vi "Dresden Edit Recipe(in).vi"() -> ()   [LabVIEW 2009] (continued)
                    n928 = local read "R Z_factor"() -> (w1701:dbl)
                    n929 = Equal To 0?(x=w1698) -> (x = 0?=w1697:bool)
                    n930 = Equal To 0?(x=w1701) -> (x = 0?=w1699:bool)
                    n931 = Equal To 0?(x=w1702) -> (x = 0?=w1700:bool)
                  }
                }
                n932 = local read "R Set Pressure mtorr"() -> (w1318:dbl)
                n933 = local read "R Argon Flow sccm"() -> (w1319:dbl)
                n934 = case shown="True" w1178 {
                  tunnel: [FALSE w1396] -> w1183
                  frame #0 {
                  }
                  frame #1 {
                    # "101"
                    n935 = local read "Calculated_total_length_dc"() -> (w1398:dbl)
                    n936 = local read "R  Total length"() -> (w1397:dbl)
                    n937 = Less?(x=w1397, y=w1398) -> (x < y?=w1396:bool)
                  }
                }
                n938 = case shown="True" w1279 {
                  tunnel: [FALSE w1388] -> w1181
                  frame #0 {
                  }
                  frame #1 {
                    # "103"
                    n939 = local read "Calculated_total_length_cmb"() -> (w1390:dbl)
                    n940 = local read "R  Total length"() -> (w1389:dbl)
                    n941 = Less?(x=w1389, y=w1390) -> (x < y?=w1388:bool)
                  }
                }
                n942 = case shown="True" w1180 {
                  tunnel: [FALSE w1392] -> w1182
                  frame #0 {
                  }
                  frame #1 {
                    # "102"
                    n943 = local read "Calculated_total_length_rf"() -> (w1394:dbl)
                    n944 = local read "R  Total length"() -> (w1393:dbl)
                    n945 = Less?(x=w1393, y=w1394) -> (x < y?=w1392:bool)
                  }
                }
                n946 = Equal To 0?(x=w1318) -> (x = 0?=w1191:bool)
                n947 = Equal To 0?(x=w1319) -> (x = 0?=w1192:bool)
                n948 = Build Array(FALSE, w1349, w1314, w1317, w1316, w1307, w1315, w1278, w1277, w1276, w1275, w1274, w1273, w1272, w1271, w1270, w1269, w1268, w1267, w1266, w1265, w1264, w1263, w1262, w1261, w1260, w1259, w1258, w1257, w1256, w1252, w1251, w1250, w1249, w1248, w1247, w1246, w1245, w1244, w1243, w1242, w1241, w1240, w1239, w1238, w1237, w1236, w1235, w1234, w1233, w1232, w1231, w1230, w1229, w1228, w1227, w1226, w1225, w1224, w1223, w1222, w1221, w1220, w1219, w1218, w1217, w1216, w1215, w1214, w1213, w1212, w1211, w1210, w1209, w1208, w1207, w1206, w1205, w1204, w1203, w1202, w1201, w1200, w1199, w1198, w1197, w1196, w1195, w1194, w1193, w1192, w1191, w1190, w1189, w1188, w1187, w1186, w1185, w1184, w1162, w1183, w1182, w1181) -> (w1255:bool[])
                n949 = Boolean To (0,1)(Boolean=w1255) -> (0, 1=w1254:i16[])
                n950 = Array Max & Min(array=w1254) -> (max index (indices)=w1253:i32)  [unwired: 3 out]
                n951 = case shown="4" w1253 {
                  tunnel: [TRUE FALSE FALSE FALSE FALSE FALSE FALSE FALSE FALSE FALSE FALSE FALSE FALSE FALSE FALSE FALSE FALSE FALSE FALSE FALSE FALSE FALSE FALSE FALSE FALSE FALSE FALSE FALSE FALSE FALSE FALSE FALSE FALSE FALSE FALSE FALSE FALSE FALSE FALSE FALSE FALSE FALSE FALSE FALSE FALSE FALSE FALSE FALSE FALSE FALSE FALSE FALSE FALSE FALSE FALSE FALSE FALSE FALSE FALSE FALSE FALSE FALSE FALSE FALSE FALSE FALSE FALSE FALSE FALSE FALSE FALSE FALSE FALSE FALSE FALSE FALSE FALSE FALSE FALSE FALSE FALSE FALSE FALSE FALSE FALSE FALSE FALSE FALSE FALSE FALSE FALSE FALSE FALSE FALSE FALSE FALSE FALSE FALSE FALSE FALSE FALSE FALSE FALSE FALSE] -> w1310
                  frame #0 {
                  }
                  frame #1 {
                    n952 = One Button Dialog(message="Please enter the Recipe name !") -> ()  [unwired: 1 in, 1 out]
                  }
                  frame #2 {
                    n953 = One Button Dialog(message="Please enter the Substrate Material name !") -> ()  [unwired: 1 in, 1 out]
                  }
                  frame #3 {
                    n954 = One Button Dialog(message="Please enter Microwave Power!") -> ()  [unwired: 1 in, 1 out]
                  }
                  frame #4 {
                    n955 = One Button Dialog(message="Please enter Pass Number !") -> ()  [unwired: 1 in, 1 out]
                  }
                  frame #5 {
                    n956 = One Button Dialog(message="Please enter Microwave Duration !") -> ()  [unwired: 1 in, 1 out]
                  }
                  frame #6 {
                    n957 = One Button Dialog(message="Please enter DC Target Material name !") -> ()  [unwired: 1 in, 1 out]
                  }
                  frame #7 {
                    n958 = One Button Dialog(message="Please click Process List!") -> ()  [unwired: 1 in, 1 out]
                  }
                  frame #8 {
                    n959 = One Button Dialog(message="Please enter DC Coating Power!") -> ()  [unwired: 1 in, 1 out]
                  }
                  frame #9 {
                    n960 = One Button Dialog(message="Please enter interval length!") -> ()  [unwired: 1 in, 1 out]
                  }
                  frame #10 {
                    n961 = One Button Dialog(message="Please enter DC Coating Power!") -> ()  [unwired: 1 in, 1 out]
                  }
                  frame #11 {
                    n962 = One Button Dialog(message="Please enter interval length!") -> ()  [unwired: 1 in, 1 out]
                  }
                  frame #12 {
                    n963 = One Button Dialog(message="Please enter DC Coating Power !") -> ()  [unwired: 1 in, 1 out]
                  }
                  frame #13 {
                    n964 = One Button Dialog(message="Please enter interval length!") -> ()  [unwired: 1 in, 1 out]
                  }
                  frame #14 {
                    n965 = One Button Dialog(message="Please enter DC Coating Power!") -> ()  [unwired: 1 in, 1 out]
                  }
                  frame #15 {
                    n966 = One Button Dialog(message="Please enter interval length!") -> ()  [unwired: 1 in, 1 out]
                  }
                  frame #16 {
                    n967 = One Button Dialog(message="Please enter DC Coating Power !") -> ()  [unwired: 1 in, 1 out]
                  }
                  frame #17 {
                    n968 = One Button Dialog(message="Please enter interval length!") -> ()  [unwired: 1 in, 1 out]
                  }
                  frame #18 {
                    n969 = One Button Dialog(message="Please enter DC Coating Power !") -> ()  [unwired: 1 in, 1 out]
                  }
                  frame #19 {
                    n970 = One Button Dialog(message="Please enter interval length!") -> ()  [unwired: 1 in, 1 out]
                  }
                  frame #20 {
                    n971 = One Button Dialog(message="Please enter DC Coating Power !") -> ()  [unwired: 1 in, 1 out]
                  }
                  frame #21 {
                    n972 = One Button Dialog(message="Please enter interval length!") -> ()  [unwired: 1 in, 1 out]
                  }
                  frame #22 {
                    n973 = One Button Dialog(message="Please enter DC Coating Power !") -> ()  [unwired: 1 in, 1 out]
                  }
                  frame #23 {
                    n974 = One Button Dialog(message="Please enter interval length!") -> ()  [unwired: 1 in, 1 out]
                  }
                  frame #24 {
                    n975 = One Button Dialog(message="Please enter DC Coating Power !") -> ()  [unwired: 1 in, 1 out]
                  }
                  frame #25 {
                    n976 = One Button Dialog(message="Please enter interval length!") -> ()  [unwired: 1 in, 1 out]
                  }
                  frame #26 {
                    n977 = One Button Dialog(message="Please enter DC Coating Power !") -> ()  [unwired: 1 in, 1 out]
                  }
                  frame #27 {
                    n978 = One Button Dialog(message="Please enter interval length!") -> ()  [unwired: 1 in, 1 out]
                  }
                  frame #28 {
                    n979 = One Button Dialog(message="Please enter RF Target Material !") -> ()  [unwired: 1 in, 1 out]
                  }
                  frame #29 {
                    n980 = One Button Dialog(message="Please click Process List!") -> ()  [unwired: 1 in, 1 out]
                  }
                  frame #30 {
                    n981 = One Button Dialog(message="Please enter RF Ramp Up Time!") -> ()  [unwired: 1 in, 1 out]
                  }
                  frame #31 {
                    n982 = One Button Dialog(message="Please enter RF Coating Power  !") -> ()  [unwired: 1 in, 1 out]
                  }
                  frame #32 {
                    n983 = One Button Dialog(message="Please enter interval length !") -> ()  [unwired: 1 in, 1 out]
                  }
                  frame #33 {
                    n984 = One Button Dialog(message="Please enter RF Coating Power  !") -> ()  [unwired: 1 in, 1 out]
                  }
                  frame #34 {
                    n985 = One Button Dialog(message="Please enter interval length!") -> ()  [unwired: 1 in, 1 out]
                  }
                  frame #35 {
                    n986 = One Button Dialog(message="Please enter RF Coating Power  !") -> ()  [unwired: 1 in, 1 out]
                  }
                  frame #36 {
                    n987 = One Button Dialog(message="Please enter interval length!") -> ()  [unwired: 1 in, 1 out]
                  }
                  frame #37 {
                    n988 = One Button Dialog(message="Please enter RF Coating Power !") -> ()  [unwired: 1 in, 1 out]
                  }
                  frame #38 {
                    n989 = One Button Dialog(message="Please enter interval length!") -> ()  [unwired: 1 in, 1 out]
                  }
                  frame #39 {
                    n990 = One Button Dialog(message="Please enter RF Coating Power !") -> ()  [unwired: 1 in, 1 out]
                  }
                  frame #40 {
                    n991 = One Button Dialog(message="Please enter interval length!") -> ()  [unwired: 1 in, 1 out]
                  }
                  frame #41 {
                    n992 = One Button Dialog(message="Please enter RF Coating Power !") -> ()  [unwired: 1 in, 1 out]
                  }
                  frame #42 {
                    n993 = One Button Dialog(message="Please enter interval length!") -> ()  [unwired: 1 in, 1 out]
                  }
                  frame #43 {
                    n994 = One Button Dialog(message="Please enter RF Coating Power !") -> ()  [unwired: 1 in, 1 out]
                  }
                  frame #44 {
                    n995 = One Button Dialog(message="Please enter interval length!") -> ()  [unwired: 1 in, 1 out]
                  }
                  frame #45 {
                    n996 = One Button Dialog(message="Please enter RF Coating Power !") -> ()  [unwired: 1 in, 1 out]
                  }
                  frame #46 {
                    n997 = One Button Dialog(message="Please enter interval length!") -> ()  [unwired: 1 in, 1 out]
                  }
                  frame #47 {
                    n998 = One Button Dialog(message="Please enter RF Coating Power !") -> ()  [unwired: 1 in, 1 out]
                  }
                  frame #48 {
                    n999 = One Button Dialog(message="Please enter interval length!") -> ()  [unwired: 1 in, 1 out]
                  }
                  frame #49 {
                    n1000 = One Button Dialog(message="Please enter RF Coating Power !") -> ()  [unwired: 1 in, 1 out]
                  }
                  frame #50 {
                    n1001 = One Button Dialog(message="Please enter interval length!") -> ()  [unwired: 1 in, 1 out]
                  }
                  frame #51 {
                    n1002 = One Button Dialog(message="Please enter RF Ramp Down Time  !") -> ()  [unwired: 1 in, 1 out]
                  }
                  frame #52 {
                    n1003 = One Button Dialog(message="Please enter Chamber II\nTarget Material name!") -> ()  [unwired: 1 in, 1 out]
                  }
                  frame #53 {
                    n1004 = One Button Dialog(message="Please enter web speed!") -> ()  [unwired: 1 in, 1 out]
                  }
                  frame #54 {
                    n1005 = One Button Dialog(message="Please enter Chamber III Target Material \nName !") -> ()  [unwired: 1 in, 1 out]
                  }
                  frame #55 {
                    n1006 = One Button Dialog(message="Please enter Web Speed !") -> ()  [unwired: 1 in, 1 out]
                  }
                  frame #56 {
                    n1007 = One Button Dialog(message="Please click process list !") -> ()  [unwired: 1 in, 1 out]
                  }
                  frame #57 {
                    n1008 = One Button Dialog(message="Please enter Number of Cycle !") -> ()  [unwired: 1 in, 1 out]
                  }
                  frame #58 {
                    n1009 = One Button Dialog(message="Please enter Chamber II  Coating Power !") -> ()  [unwired: 1 in, 1 out]
                  }
                  frame #59 {
                    n1010 = One Button Dialog(message="Please enter Chamber III  Coating Power !") -> ()  [unwired: 1 in, 1 out]
                  }
                  frame #60 {
                    n1011 = One Button Dialog(message="Please enter interval length!") -> ()  [unwired: 1 in, 1 out]
                  }
                  frame #61 {
                    n1012 = One Button Dialog(message="Please enter Chamber II  Coating Power !") -> ()  [unwired: 1 in, 1 out]
                  }
                  frame #62 {
                    n1013 = One Button Dialog(message="Please enter Chamber III  Coating Power !") -> ()  [unwired: 1 in, 1 out]
                  }
                  frame #63 {
                    n1014 = One Button Dialog(message="Please enter interval length!") -> ()  [unwired: 1 in, 1 out]
                  }
                  frame #64 {
                    n1015 = One Button Dialog(message="Please enter Chamber II  Coating Power !") -> ()  [unwired: 1 in, 1 out]
                  }
                  frame #65 {
                    n1016 = One Button Dialog(message="Please enter Chamber III Coating Power !") -> ()  [unwired: 1 in, 1 out]
                  }
                  frame #66 {
                    n1017 = One Button Dialog(message="Please enter interval length!") -> ()  [unwired: 1 in, 1 out]
                  }
                  frame #67 {
                    n1018 = One Button Dialog(message="Please enter Chamber II  Coating Power !") -> ()  [unwired: 1 in, 1 out]
                  }
                  frame #68 {
                    n1019 = One Button Dialog(message="Please enter Chamber III  Coating Power !") -> ()  [unwired: 1 in, 1 out]
                  }
                  frame #69 {
                    n1020 = One Button Dialog(message="Please enter interval length!") -> ()  [unwired: 1 in, 1 out]
                  }
                  frame #70 {
                    n1021 = One Button Dialog(message="Please enter Chamber II  Coating Power !") -> ()  [unwired: 1 in, 1 out]
                  }
                  frame #71 {
                    n1022 = One Button Dialog(message="Please enter Chamber III  Coating Power !") -> ()  [unwired: 1 in, 1 out]
                  }
                  frame #72 {
                    n1023 = One Button Dialog(message="Please enter interval length!") -> ()  [unwired: 1 in, 1 out]
                  }
                  frame #73 {
                    n1024 = One Button Dialog(message="Please enter Chamber II  Coating Power !") -> ()  [unwired: 1 in, 1 out]
                  }
                  frame #74 {
                    n1025 = One Button Dialog(message="Please enter Chamber III  Coating Power !") -> ()  [unwired: 1 in, 1 out]
                  }
                  frame #75 {
                    n1026 = One Button Dialog(message="Please enter interval length!") -> ()  [unwired: 1 in, 1 out]
                  }
                  frame #76 {
                    n1027 = One Button Dialog(message="Please enter Chamber II  Coating Power !") -> ()  [unwired: 1 in, 1 out]
                  }
                  frame #77 {
                    n1028 = One Button Dialog(message="Please enter Chamber III  Coating Power !") -> ()  [unwired: 1 in, 1 out]
                  }
                  frame #78 {
                    n1029 = One Button Dialog(message="Please enter interval length!") -> ()  [unwired: 1 in, 1 out]
                  }
                  frame #79 {
                    n1030 = One Button Dialog(message="Please enter Chamber II  Coating Power !") -> ()  [unwired: 1 in, 1 out]
                  }
                  frame #80 {
                    n1031 = One Button Dialog(message="Please enter Chamber III  Coating Power !") -> ()  [unwired: 1 in, 1 out]
                  }
                  frame #81 {
                    n1032 = One Button Dialog(message="Please enter interval length!") -> ()  [unwired: 1 in, 1 out]
                  }
                  frame #82 {
                    n1033 = One Button Dialog(message="Please enter Chamber II  Coating Power !") -> ()  [unwired: 1 in, 1 out]
                  }
                  frame #83 {
                    n1034 = One Button Dialog(message="Please enter Chamber III  Coating Power !") -> ()  [unwired: 1 in, 1 out]
                  }
                  frame #84 {
                    n1035 = One Button Dialog(message="Please enter interval length!") -> ()  [unwired: 1 in, 1 out]
                  }
                  frame #85 {
                    n1036 = One Button Dialog(message="Please enter Chamber II  Coating Power !") -> ()  [unwired: 1 in, 1 out]
                  }
                  frame #86 {
                    n1037 = One Button Dialog(message="Please enter Chamber III  Coating Power !") -> ()  [unwired: 1 in, 1 out]
                  }
                  frame #87 {
                    n1038 = One Button Dialog(message="Please enter interval length!") -> ()  [unwired: 1 in, 1 out]
                  }
                  frame #88 {
                    n1039 = One Button Dialog(message="Please enter Material Density !") -> ()  [unwired: 1 in, 1 out]
                  }
                  frame #89 {
                    n1040 = One Button Dialog(message="Please enter Z factor !") -> ()  [unwired: 1 in, 1 out]
                  }
                  frame #90 {
                    n1041 = One Button Dialog(message="Please enter Tooling Factor !") -> ()  [unwired: 1 in, 1 out]
                  }
                  frame #91 {
                    n1042 = One Button Dialog(message="Please enter Argon Flow !") -> ()  [unwired: 1 in, 1 out]
                  }
                  frame #92 {
                    n1043 = One Button Dialog(message="Please enter Set Pressure !") -> ()  [unwired: 1 in, 1 out]
                  }
                  frame #93 {
                    n1044 = One Button Dialog(message="Please enter Target thickness Value!") -> ()  [unwired: 1 in, 1 out]
                  }
                  frame #94 {
                    n1045 = One Button Dialog(message="Please enter Duration!") -> ()  [unwired: 1 in, 1 out]
                  }
                  frame #95 {
                    n1046 = One Button Dialog(message="Please enter Minimum Diameter !") -> ()  [unwired: 1 in, 1 out]
                  }
                  frame #96 {
                    n1047 = One Button Dialog(message="Please enter Maximum Diameter !") -> ()  [unwired: 1 in, 1 out]
                  }
                  frame #97 {
                    n1048 = One Button Dialog(message="Please enter Web Speed !") -> ()  [unwired: 1 in, 1 out]
                  }
                  frame #98 {
                    n1049 = One Button Dialog(message="Please enter Web Thickness !") -> ()  [unwired: 1 in, 1 out]
                  }
                  frame #99 {
                    n1050 = One Button Dialog(message="Please enter Tension Value !") -> ()  [unwired: 1 in, 1 out]
                  }
                  frame #100 {
                    n1051 = One Button Dialog(message="Please click equal sign!") -> ()  [unwired: 1 in, 1 out]
                  }
                  frame #101 {
                    n1052 = One Button Dialog(message="Total length is not enough for process !") -> ()  [unwired: 1 in, 1 out]
                  }
                  frame #102 {
                    n1053 = One Button Dialog(message="Total length is not enough for process !") -> ()  [unwired: 1 in, 1 out]
                  }
                  frame #103 {
                    n1054 = One Button Dialog(message="Total length is not enough for process !") -> ()  [unwired: 1 in, 1 out]
                  }
                }
              }
            }
            n1055 = case shown="True" w859 {
              frame #0 {
              }
              frame #1 {
                n1056 = local read "R_Thickness Selection"() -> (w1915:enum32{"Thickness", "Time"})
                n1057 = case shown="\"Time\"" w1915 {
                  frame #0 {
                    n1058 = local write "R_Duration"(0.0 ("R_Duration")) -> ()
                    n1059 = property on="R_Target Thickness Value" class="DigNum (strict)"("DisabledEnum"=T5."Enabled" ("Disabled")) -> ()  [unwired: 2 in, 2 out]
                    n1060 = property on="R_Duration" class="DigNum (strict)"("DisabledEnum"=T5."Disabled and Grayed Out" ("Disabled")) -> ()  [unwired: 2 in, 2 out]
                  }
                  frame #1 {
                    n1061 = local write "R_Target Thickness Value"(0.0 ("R_Target Thickness Value")) -> ()
                    n1062 = property on="R_Target Thickness Value" class="DigNum (strict)"("DisabledEnum"=T5."Disabled and Grayed Out" ("Disabled")) -> ()  [unwired: 2 in, 2 out]
                    n1063 = property on="R_Duration" class="DigNum (strict)"("DisabledEnum"=T5."Enabled" ("Disabled")) -> ()  [unwired: 2 in, 2 out]
                  }
                }
              }
            }
            n1064 = case shown="True" w856 {
              frame #0 {
                n1065 = property on="R_Thickness Selection" class="RadioBtnsControl (strict)"("DisabledEnum"=T5."Enabled" ("Disabled")) -> ()  [unwired: 2 in, 2 out]
              }
              frame #1 {
                w1913 = T5."Disabled and Grayed Out" ("Disabled")
                n1066 = local write "R_Duration"(0.0 ("R_Duration")) -> ()
                n1067 = local write "R_Target Thickness Value"(0.0 ("R_Target Thickness Value")) -> ()
                n1068 = property on="R_Target Thickness Value" class="DigNum (strict)"("DisabledEnum"=T5."Disabled and Grayed Out" ("Disabled")) -> ()  [unwired: 2 in, 2 out]
                n1069 = property on="R_Thickness Selection" class="RadioBtnsControl (strict)"("DisabledEnum"=w1913) -> ()  [unwired: 2 in, 2 out]
                n1070 = property on="R_Duration" class="DigNum (strict)"("DisabledEnum"=w1913) -> ()  [unwired: 2 in, 2 out]
              }
            }
            n1071 = case shown="False" w996 {
              frame #0 {
                n1072 = local write "R Single RF Ramp down Time"(0.0 ("Target Clean Power")) -> ()
                n1073 = property on="R Single RF Ramp down Time" class="DigNum (strict)"("DisabledEnum"=T5."Disabled and Grayed Out" ("Disabled")) -> ()  [unwired: 2 in, 2 out]
              }
              frame #1 {
                n1074 = property on="R Single RF Ramp down Time" class="DigNum (strict)"("DisabledEnum"=T5."Enabled" ("Disabled")) -> ()  [unwired: 2 in, 2 out]
              }
            }
            n1075 = case shown="\"Combination Sputter\"" w1006 {
              frame #0 {
                n1076 = local write "Recipe_selection tab"(0) -> ()
              }
              frame #1 {
                n1077 = local write "Recipe_selection tab"(1) -> ()
              }
            }
            n1078 = case shown="\"Other\"" w1010 {
              frame #0 {
                n1079 = local write "Web_selection_tab"(0) -> ()
              }
              frame #1 {
                n1080 = local write "Web_selection_tab"(1) -> ()
              }
            }
            n1081 = case shown="\"RF Sputter\"" w1005 {
              frame #0 {
                n1082 = local write "R_Single_Coating Type Selection_tab"(0) -> ()
              }
              frame #1 {
                n1083 = local write "R_Single_Coating Type Selection_tab"(1) -> ()
              }
              frame #2 {
                n1084 = local write "R_Single_Coating Type Selection_tab"(2) -> ()
              }
            }
            n1085 = case shown="False" w997 {
              frame #0 {
                w2458 = T5."Disabled and Grayed Out" ("Disabled")
                w2457 = 0.0 ("Target Clean Power")
                n1086 = local write "R Single RF  Step1 Coating Power"(w2457) -> ()
                n1087 = local write "R Single RF Interval length"(w2457) -> ()
                n1088 = property on="R Single RF  Step1 Coating Power" class="DigNum (strict)"("DisabledEnum"=w2458) -> ()  [unwired: 2 in, 2 out]
                n1089 = property on="R Single RF Interval length" class="DigNum (strict)"("DisabledEnum"=w2458) -> ()  [unwired: 2 in, 2 out]
              }
              frame #1 {
                w2459 = T5."Enabled" ("Disabled")
                n1090 = property on="R Single RF  Step1 Coating Power" class="DigNum (strict)"("DisabledEnum"=w2459) -> ()  [unwired: 2 in, 2 out]
                n1091 = property on="R Single RF Interval length" class="DigNum (strict)"("DisabledEnum"=w2459) -> ()  [unwired: 2 in, 2 out]
              }
            }
            n1092 = case shown="True" w995 {
              frame #0 {
                n1093 = local write "R Single RF Ramp up Time"(0.0 ("Target Clean Power")) -> ()
                n1094 = property on="R Single RF Ramp up Time" class="DigNum (strict)"("DisabledEnum"=T5."Disabled and Grayed Out" ("Disabled")) -> ()  [unwired: 2 in, 2 out]
              }
              frame #1 {
                n1095 = property on="R Single RF Ramp up Time" class="DigNum (strict)"("DisabledEnum"=T5."Enabled" ("Disabled")) -> ()  [unwired: 2 in, 2 out]
              }
            }
            n1096 = case shown="False" w998 {
              frame #0 {
                w2463 = 0.0 ("Ramp up Time")
                w2464 = T5."Disabled and Grayed Out" ("Disabled")
                n1097 = local write "R Single DC Step1 Coating Power"(w2463) -> ()
                n1098 = local write "R Single DC Interval length1"(w2463) -> ()
                n1099 = property on="R Single DC Step1 Coating Power" class="DigNum (strict)"("DisabledEnum"=w2464) -> ()  [unwired: 2 in, 2 out]
                n1100 = property on="R Single DC Interval length1" class="DigNum (strict)"("DisabledEnum"=w2464) -> ()  [unwired: 2 in, 2 out]
              }
              frame #1 {
                w2465 = T5."Enabled" ("Disabled")
                n1101 = property on="R Single DC Interval length1" class="DigNum (strict)"("DisabledEnum"=w2465) -> ()  [unwired: 2 in, 2 out]
                n1102 = property on="R Single DC Step1 Coating Power" class="DigNum (strict)"("DisabledEnum"=w2465) -> ()  [unwired: 2 in, 2 out]
              }
            }
            n1103 = local read "R Single DC Interval length1"() -> (w959:dbl)
            n1104 = Boolean To (0,1)(Boolean=w973) -> (0, 1=w972:i16)
            n1105 = Boolean To (0,1)(Boolean=w981) -> (0, 1=w980:i16)
            n1106 = Boolean To (0,1)(Boolean=w979) -> (0, 1=w978:i16)
            n1107 = local read "R Single DC Interval length2"() -> (w958:dbl)
            n1108 = Boolean To (0,1)(Boolean=w965) -> (0, 1=w971:i16)
            n1109 = Boolean To (0,1)(Boolean=w964) -> (0, 1=w970:i16)
            n1110 = Boolean To (0,1)(Boolean=w975) -> (0, 1=w974:i16)
            n1111 = local read "R Single DC Interval length3"() -> (w957:dbl)
            n1112 = Boolean To (0,1)(Boolean=w963) -> (0, 1=w969:i16)
            n1113 = Boolean To (0,1)(Boolean=w962) -> (0, 1=w968:i16)
            n1114 = local read "R Single DC Interval length4"() -> (w956:dbl)
            n1115 = local read "R Single DC Interval length5"() -> (w955:dbl)
            n1116 = Boolean To (0,1)(Boolean=w961) -> (0, 1=w967:i16)
            n1117 = local read "R Single DC Interval length6"() -> (w954:dbl)
            n1118 = local read "R Single DC Interval length8"() -> (w952:dbl)
            n1119 = local read "R Single DC Interval length7"() -> (w953:dbl)
            n1120 = Boolean To (0,1)(Boolean=w960) -> (0, 1=w966:i16)
            n1121 = local read "R Single DC Interval length9"() -> (w951:dbl)
            n1122 = local read "R Single DC Interval length10"() -> (w950:dbl)
            n1123 = local read "R Single RF Interval length2"() -> (w920:dbl)
            n1124 = local read "R Single RF Interval length3"() -> (w919:dbl)
            n1125 = local read "R Single RF Interval length"() -> (w921:dbl)
            n1126 = Boolean To (0,1)(Boolean=w930) -> (0, 1=w939:i16)
            n1127 = local read "R Single RF Interval length4"() -> (w918:dbl)
            n1128 = Boolean To (0,1)(Boolean=w927) -> (0, 1=w936:i16)
            n1129 = Boolean To (0,1)(Boolean=w926) -> (0, 1=w935:i16)
            n1130 = Boolean To (0,1)(Boolean=w925) -> (0, 1=w934:i16)
            n1131 = Boolean To (0,1)(Boolean=w929) -> (0, 1=w938:i16)
            n1132 = local read "R Single RF Interval length5"() -> (w917:dbl)
            n1133 = local read "R Single RF Interval length8"() -> (w914:dbl)
            n1134 = Boolean To (0,1)(Boolean=w928) -> (0, 1=w937:i16)
            n1135 = Boolean To (0,1)(Boolean=w923) -> (0, 1=w932:i16)
            n1136 = Boolean To (0,1)(Boolean=w924) -> (0, 1=w933:i16)
            n1137 = local read "R Single RF Interval length7"() -> (w915:dbl)
            n1138 = Boolean To (0,1)(Boolean=w922) -> (0, 1=w931:i16)
            n1139 = local read "R Single RF Interval length10"() -> (w912:dbl)
            n1140 = local read "R Single RF Interval length6"() -> (w916:dbl)
            n1141 = Boolean To (0,1)(Boolean=w940) -> (0, 1=w941:i16)
            n1142 = local read "R Single RF Interval length9"() -> (w913:dbl)
            n1143 = Multiply(x=w980, y=w959) -> (x*y=w977:dbl)
            n1144 = Multiply(x=w978, y=w958) -> (x*y=w976:dbl)
            n1145 = Multiply(x=w974, y=w957) -> (x*y=w949:dbl)
            n1146 = Multiply(x=w972, y=w956) -> (x*y=w948:dbl)
            n1147 = Multiply(x=w971, y=w955) -> (x*y=w947:dbl)
            n1148 = Multiply(x=w970, y=w954) -> (x*y=w945:dbl)
            n1149 = Multiply(x=w969, y=w953) -> (x*y=w946:dbl)
            n1150 = Multiply(x=w968, y=w952) -> (x*y=w944:dbl)
            n1151 = Multiply(x=w939, y=w920) -> (x*y=w910:dbl)
            n1152 = Multiply(x=w936, y=w917) -> (x*y=w907:dbl)
            n1153 = Multiply(x=w935, y=w916) -> (x*y=w906:dbl)
            n1154 = Multiply(x=w934, y=w915) -> (x*y=w905:dbl)
            n1155 = Multiply(x=w938, y=w919) -> (x*y=w909:dbl)
            n1156 = Multiply(x=w967, y=w951) -> (x*y=w943:dbl)
            n1157 = Multiply(x=w937, y=w918) -> (x*y=w908:dbl)
            n1158 = Multiply(x=w932, y=w913) -> (x*y=w903:dbl)
            n1159 = Multiply(x=w933, y=w914) -> (x*y=w904:dbl)
            n1160 = Multiply(x=w931, y=w912) -> (x*y=w902:dbl)
            n1161 = Multiply(x=w966, y=w950) -> (x*y=w942:dbl)
            n1162 = Multiply(x=w941, y=w921) -> (x*y=w911:dbl)
            n1163 = local read "R_Simple_Coating Type Selection"() -> (w1004:T2)
            n1164 = local read "R_Simple_Coating Type Selection"() -> (w1003:T2)
            n1165 = Compound Arithmetic op=ADD(w977, w976, w949, w948, w947, w945, w946, w944, w943, w942) -> (→"Calculated_total_length_dc":dbl)
            n1166 = Compound Arithmetic op=ADD(w911, w910, w909, w908, w907, w906, w905, w904, w903, w902) -> (→"Calculated_total_length_rf":dbl)
            n1167 = local read "R Single DC Step9 Coating Power Active"() -> (w842:bool)
            n1168 = local read "R Single DC Step8 Coating Power Active"() -> (w843:bool)
            n1169 = local read "R Cmb Step1 Coating Power Active"() -> (w890:bool)
            n1170 = local read "R_Simple_Coating Type Selection"() -> (w1002:T2)
            n1171 = local read "R_Recipe_type_selection"() -> (w1001:enum32{"Single Recipe", "Combination Sputter"})
            n1172 = Equal?(x=w1004, y=0) -> (x = y?=w1016:bool)
            n1173 = Equal?(x=w1002, y=2) -> (x = y?=w1011:bool)
            n1174 = Equal?(x=w1003, y=1) -> (x = y?=w1013:bool)
            n1175 = local read "Thickness_Monitor_Active"() -> (w988:bool)
            n1176 = local read "R Cmb Step2 Coating Power Active"() -> (w888:bool)
